vi "VI_ParseELOG-FetchString.vi"(5 "TimestampIncluded":bool, 7 "NumOfCalcModes":i32, 8 "error in (no error)":errorcluster, 10 "FetchDataString":string="0.1, 1.5, 1, 10.5, 10, 0.2, 2.5, 2, 20.5, 20, 0.3, 3.5, 3, 30.5, 30", 11 "Common Refs":T1={"LBox_ChList"=refnum, "STR_LoggingChName1"=refnum, "Listbox_ChValue"=refnum, "STR_LoggingChName2"=refnum, "STR_LoggingChName3"=refnum, "STR_LoggingChName4"=refnum, "STR_LoggingChName5"=refnum, "STR_LoggingChName6"=refnum, "OXY_SCPI Ref"="TCPIP0::192.168.1.75::10001::SOCKET", "STR_ChName1"=refnum, "STR_ChName2"=refnum, "STR_ChName3"=refnum, "STR_ChName4"=refnum, "STR_ChName5"=refnum, "STR_ChName6"=refnum, "Enum_SelectTimestampFormat"=refnum, "GRAPH-XY_ELOG"=refnum, "GRAPH-XY_Measurement"=refnum, "Button_StartBuffer"=refnum, "Button_StopBuffer"=refnum, "Button_FetchData"=refnum, "STR_LoggingChName1"=refnum, "STR_LoggingChName2"=refnum, "STR_LoggingChName3"=refnum, "STR_LoggingChName4"=refnum, "STR_LoggingChName5"=refnum, "STR_LoggingChName6"=refnum, "Enum_SelectCalc"=refnum, "Num_SetDurationTime"=refnum, "Button_StopTransfer"=refnum, "Button_StartTransfer"=refnum, "STR_IN_AggregationRate"=refnum, "Button_Disconnect"=refnum, "Button_Connect"=refnum, "Button_StartRec"=refnum, "Button_PauseRec"=refnum, "Button_StopRec"=refnum, "Bool_StatusLED"=refnum, "Indicator_RecordingStatus"=refnum}) -> (0 "error out":errorcluster, 1 "Corrected_LoggingChName":string[](array[string]), 2 "Fomarted List":string[][][](array[string]), 3 "Timestamp only list":string[](array[string]))   [LabVIEW 2018]
uses:
  TypeDefs/Refs_Common.ctl
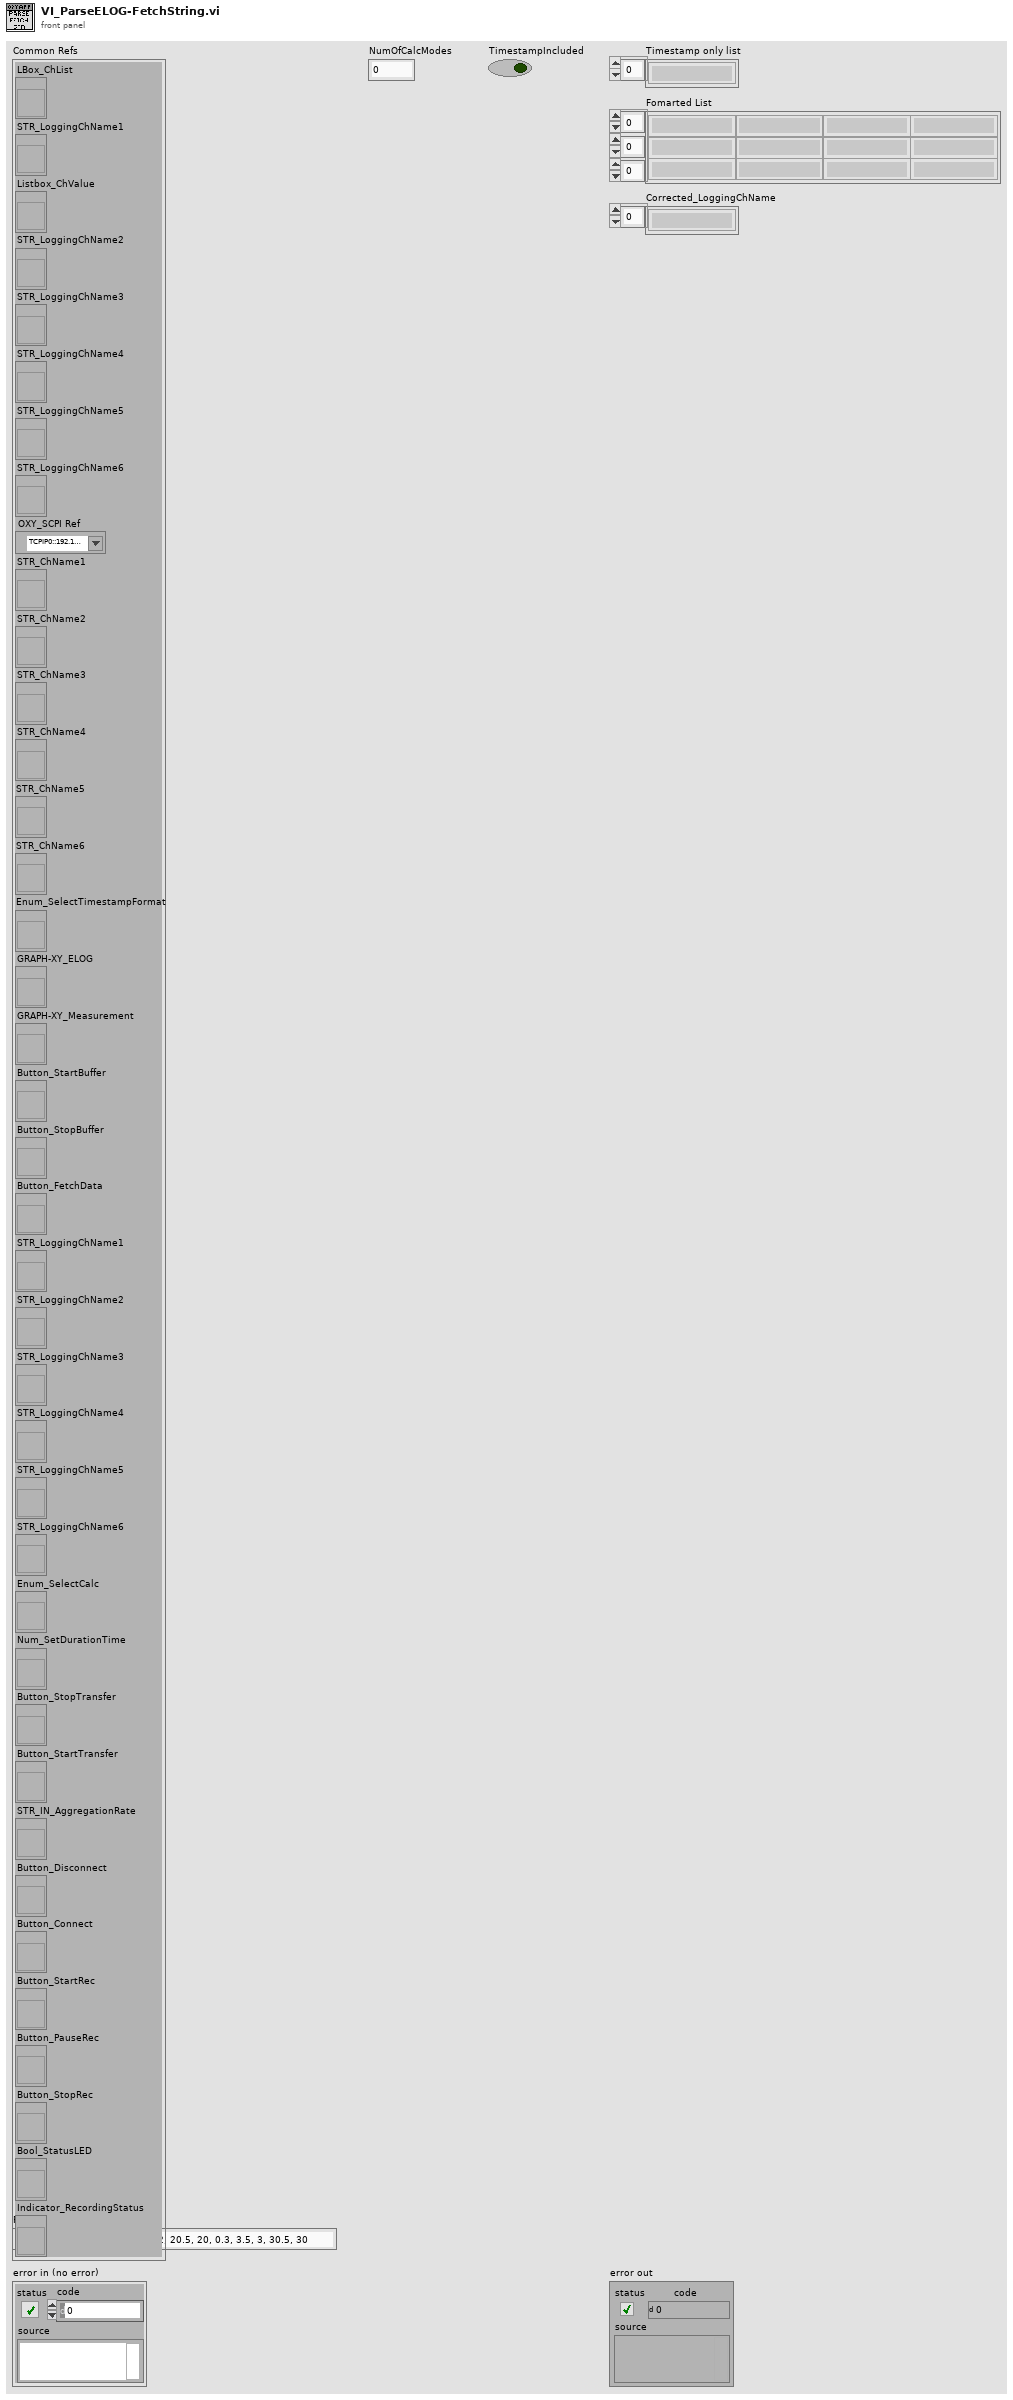
[diagram p1: front panel]
types:
  T1 = typedef "Refs_Common.ctl" = cluster{"LBox_ChList":refnum<vi>, "STR_LoggingChName1":refnum<vi>, "Listbox_ChValue":refnum<vi>, "STR_LoggingChName2":refnum<vi>, "STR_LoggingChName3":refnum<vi>, "STR_LoggingChName4":refnum<vi>, "STR_LoggingChName5":refnum<vi>, "STR_LoggingChName6":refnum<vi>, "OXY_SCPI Ref":refnum<visa-resource-name>, "STR_ChName1":refnum<vi>, "STR_ChName2":refnum<vi>, "STR_ChName3":refnum<vi>, "STR_ChName4":refnum<vi>, "STR_ChName5":refnum<vi>, "STR_ChName6":refnum<vi>, "Enum_SelectTimestampFormat":refnum<vi>, "GRAPH-XY_ELOG":refnum<vi>, "GRAPH-XY_Measurement":refnum<vi>, "Button_StartBuffer":refnum<vi>, "Button_StopBuffer":refnum<vi>, "Button_FetchData":refnum<vi>, "STR_LoggingChName1":refnum<vi>, "STR_LoggingChName2":refnum<vi>, "STR_LoggingChName3":refnum<vi>, "STR_LoggingChName4":refnum<vi>, "STR_LoggingChName5":refnum<vi>, "STR_LoggingChName6":refnum<vi>, "Enum_SelectCalc":refnum<vi>, "Num_SetDurationTime":refnum<vi>, "Button_StopTransfer":refnum<vi>, "Button_StartTransfer":refnum<vi>, "STR_IN_AggregationRate":refnum<vi>, "Button_Disconnect":refnum<vi>, "Button_Connect":refnum<vi>, "Button_StartRec":refnum<vi>, "Button_PauseRec":refnum<vi>, "Button_StopRec":refnum<vi>, "Bool_StatusLED":refnum<vi>, "Indicator_RecordingStatus":refnum<vi>}
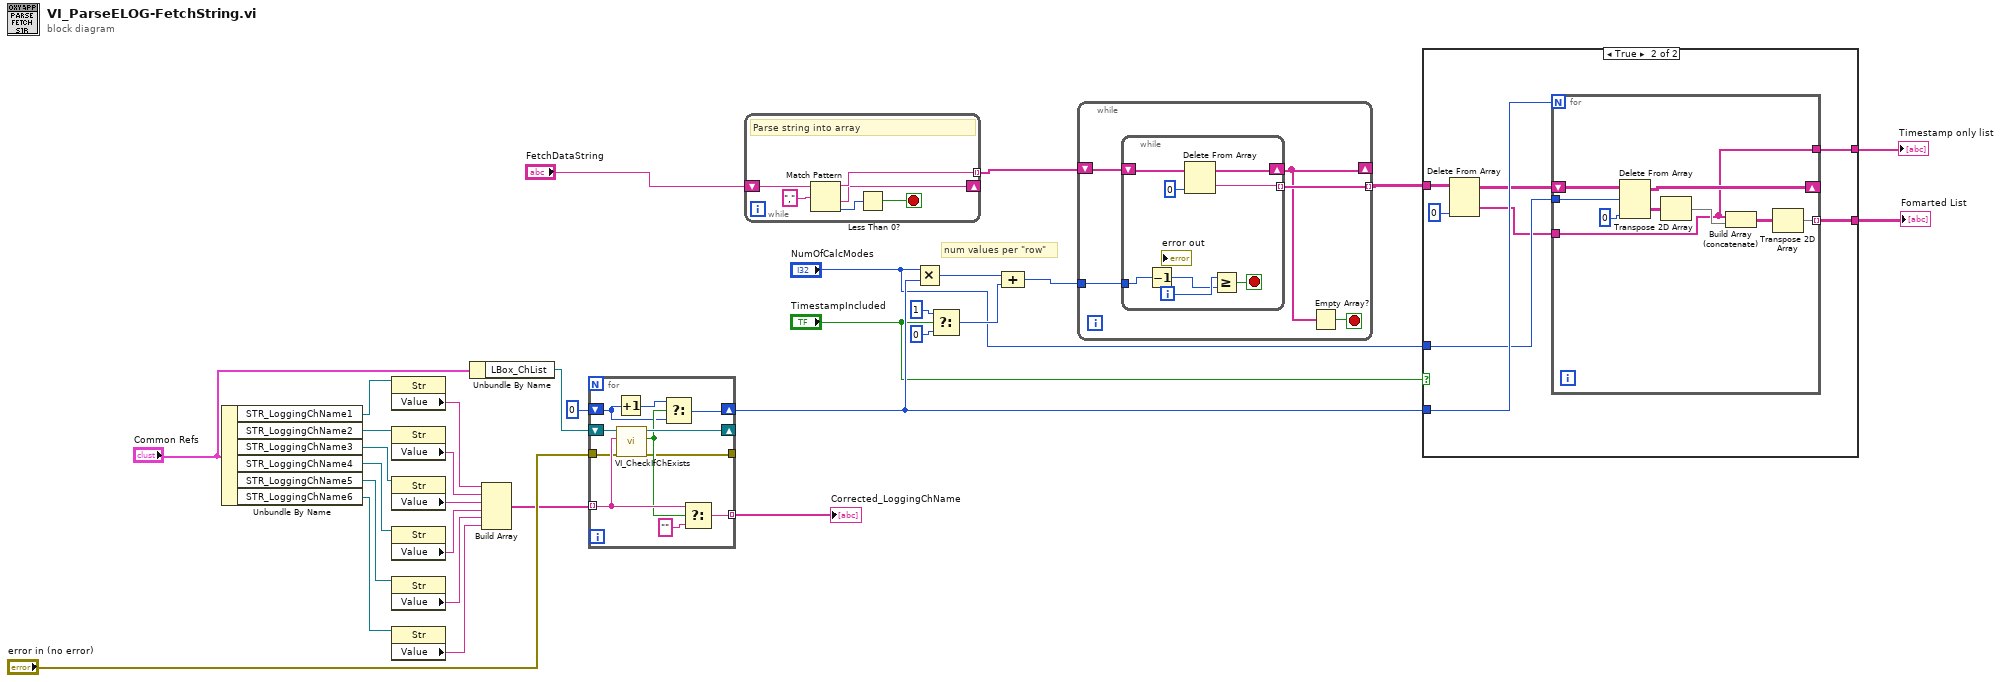
[diagram p0: block diagram]
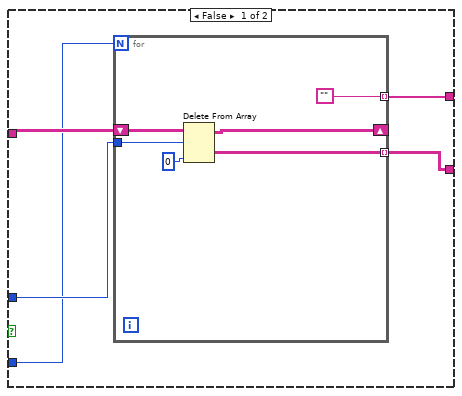
[diagram p2: hidden frame]
diagram:
  # "num values per \"row\""
  n1 = Unbundle By Name("Common Refs") -> ("STR_LoggingChName1"=w17:refnum<vi>, "STR_LoggingChName2"=w16:refnum<vi>, "STR_LoggingChName3"=w15:refnum<vi>, "STR_LoggingChName4"=w14:refnum<vi>, "STR_LoggingChName5"=w13:refnum<vi>, "STR_LoggingChName6"=w12:refnum<vi>)
  n2 = property class="Str"(reference=w17) -> ("Value"=w11:string)  [unwired: 1 in, 2 out]
  n3 = property class="Str"(reference=w16) -> ("Value"=w10:string)  [unwired: 1 in, 2 out]
  n4 = property class="Str"(reference=w15) -> ("Value"=w9:string)  [unwired: 1 in, 2 out]
  n5 = property class="Str"(reference=w14) -> ("Value"=w8:string)  [unwired: 1 in, 2 out]
  n6 = property class="Str"(reference=w13) -> ("Value"=w7:string)  [unwired: 1 in, 2 out]
  n7 = property class="Str"(reference=w12) -> ("Value"=w6:string)  [unwired: 1 in, 2 out]
  n8 = Unbundle By Name("Common Refs") -> ("LBox_ChList"=w4:refnum<vi>)
  n9 = Build Array(w11, w10, w9, w8, w7, w6) -> (w5:string[])
  n10 = for {
    tunnel: w5 -> [w40] mode=indexing
    shift-right: [w41] -> _
    shift-left: w4 -> [w42]
    tunnel: [w38] -> w28 mode=indexing
    shift-right: [w34] -> w23
    shift-left: 0 -> [w35]
    tunnel: "error in (no error)" -> [w33]
    tunnel: [w32] -> _
    n11 = Increment(x=w35) -> (x+1=w36:i32)
    n12 = call "VI_CheckIfChExists.vi"("error in (no error)"=w33, "Channel Name To Check"=w40, "ChList_Ref In"=w42) -> ("error out"=w32:errorcluster, "Channel Exists"=w37:bool, "ChList_Ref Out"=w41:refnum<vi>)  [unwired: 6 in]
    n13 = Select(t=w36, s=w37, f=w35) -> (s? t:f=w34:i32)
    n14 = Select(t=w40, s=w37, f="") -> (s? t:f=w38:string)
  }
  "Corrected_LoggingChName" <- w28
  n15 = while {
    shift-right: [w43] -> _
    shift-left: "FetchDataString" -> [w47]
    tunnel: [w44] -> w24 mode=indexing
    stop <- w45 stop-if-true
    # "Parse string into array"
    n16 = Match Pattern(string=w47, regular expression=",") -> (before substring=w44:string, after substring=w43:string, offset past match=w46:i32)  [unwired: 1 in, 1 out]
    n17 = Less Than 0?(x=w46) -> (x < 0?=w45:bool)
  }
  n18 = Multiply(x="NumOfCalcModes", y=w23) -> (x*y=w27:i32)
  n19 = Select(t=1, s="TimestampIncluded", f=0) -> (s? t:f=w26:i32)
  n20 = Compound Arithmetic op=ADD(w27, w26) -> (w25:i32)
  n21 = while {
    tunnel: w25 -> [w53]
    tunnel: [w52] -> w22 mode=indexing
    shift-right: [w49] -> _
    shift-left: w24 -> [w51]
    stop <- w50 stop-if-true
    n22 = while {
      tunnel: w53 -> [w55]
      tunnel: [w57] -> w52 mode=indexing
      shift-right: [w56] -> w49
      shift-left: w51 -> [w59]
      i -> [w61]
      stop <- w60 stop-if-true
      n23 = Decrement(x=w55) -> (x-1=w54:i32)
      n24 = Delete From Array(array=w59, index=0) -> (deleted portion=w57:string, array with subset deleted=w56:string[])  [unwired: 1 in]
      n25 = Greater Or Equal?(x=w61, y=w54) -> (x >= y?=w60:bool)
    }
    n26 = Empty Array?(array=w49) -> (empty?=w50:bool)
  }
  n27 = case shown="True" "TimestampIncluded" {
    tunnel: w23 -> [w63 w80]
    tunnel: w22 -> [w66 w79]
    tunnel: "NumOfCalcModes" -> [w65 w76]
    tunnel: [w64 w74] -> w20
    tunnel: [w62 w73] -> w1
    frame False {
      n28 = for {
        N: w63 -> [_]
        shift-right: [w69] -> _
        shift-left: w66 -> [w71]
        tunnel: w65 -> [w70]
        tunnel: [w68] -> w64 mode=indexing
        tunnel: [""] -> w62 mode=indexing
        n29 = Delete From Array(array=w71, length=w70, index (col)=0 ("disabled index (col)")) -> (deleted portion=w68:string[][], array with subset deleted=w69:string[][])  [unwired: 1 in]
      }
    }
    frame True {
      n30 = Delete From Array(array=w79, index (col)=0 ("disabled index (col)")) -> (deleted portion=w75:string[], array with subset deleted=w77:string[][])  [unwired: 2 in]
      n31 = for {
        N: w80 -> [_]
        shift-right: [w86] -> _
        shift-left: w77 -> [w88]
        tunnel: w76 -> [w87]
        tunnel: w75 -> [w81]
        tunnel: [w85] -> w74 mode=indexing
        tunnel: [w81] -> w73
        n32 = Delete From Array(array=w88, length=w87, index (col)=0 ("disabled index (col)")) -> (deleted portion=w82:string[][], array with subset deleted=w86:string[][])  [unwired: 1 in]
        n33 = Transpose 2D Array(2D array=w82) -> (transposed array=w83:string[][])
        n34 = Build Array (concatenate)(w81, w83) -> (w84:string[][])
        n35 = Transpose 2D Array(2D array=w84) -> (transposed array=w85:string[][])
      }
    }
  }
  "Fomarted List" <- w20
  "Timestamp only list" <- w1
